vi "To XML (Core).vi"(8 "error in (no error)":errorcluster, 10 "Parent":refnum<k20>, 11 "Property in":refnum<class "Property.lvclass">) -> (0 "error out":errorcluster)   [LabVIEW 2013, in "JUnit XML.lvlib" / "Property.lvclass"]
doc: "Serializes a Property using NI XML Parser."
uses:
  Property.lvclass
  Property.lvclass/Property.ctl
  <vilib>/xml/Close Reference(Node).vi
  <vilib>/xml/NI_XML.lvlib
  JUnit XML.lvlib
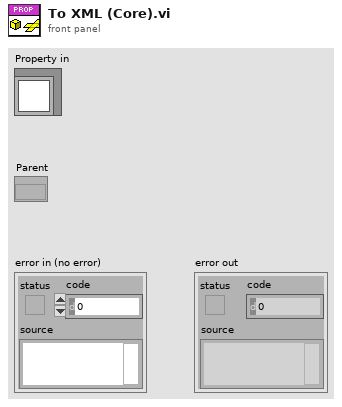
[diagram p1: front panel]
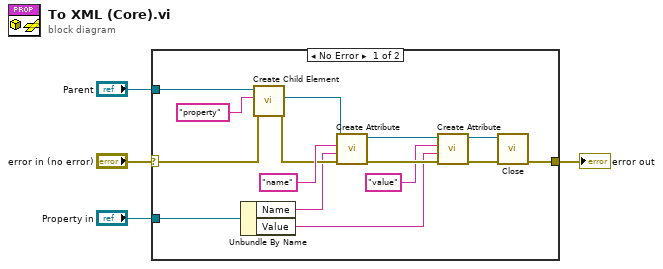
[diagram p0: block diagram]
diagram:
  n1 = case shown="No Error" "error in (no error)" {
    selector: "error in (no error)" -> [w9 w20]
    tunnel: [w8 w20] -> w3
    tunnel: "Property in" -> [w7 _]
    tunnel: "Parent" -> [w10 _]
    frame No Error {
      n2 = Unbundle By Name(w7) -> ("Name"=w6:string, "Value"=w5:string)
      n3 = call "Create Child Element.vi"("error in (no error)"=w9, "Name"="property" ("Tag Name"), "Node in"=w10) -> ("error out"=w13:errorcluster, "Child Element"=w14:refnum<k20>)  [unwired: 6 in, 1 out]
      n4 = call "Create Attribute.vi"("error in (no error)"=w13, "Value"=w6, "Name"="name" ("Attribute Name"), "Element in"=w14) -> ("error out"=w16:errorcluster, "Element out"=w17:refnum<k20>)  [unwired: 6 in]
      n5 = call "Create Attribute.vi"("error in (no error)"=w16, "Value"=w5, "Name"="value" ("Attribute Name"), "Element in"=w17) -> ("error out"=w11:errorcluster, "Element out"=w12:refnum<k20>)  [unwired: 6 in]
      n6 = call-poly <vilib>:"Close.vi"("error in (no error)"=w11, "node"=w12) -> ("error out"=w8:errorcluster)  [unwired: 7 in]
    }
    frame Error {
    }
  }
  "error out" <- w3
